vi "test Diff Configuration (Add Remove Ports and Acyclic Frame).vi"(8 "error in":errorcluster, 11 "TestCase in":refnum<class "Refresh.lvclass">) -> (0 "error out":errorcluster, 3 "TestCase out":refnum<class "Refresh.lvclass">)   [LabVIEW 2020, in "Refresh.lvclass"]
uses:
  Refresh.lvclass
  <vilib>/addons/_JKI Toolkits/VI Tester/TestCase.llb/TestCase.lvclass
  System Explorer/Implementation/System Explorer/Refresh/Refresh.lvlib
  Shared/Parameter Definition.ctl
  Shared/Address.ctl
  Shared/Terminal Endpoint.ctl
  Shared/Message Type.ctl
  Shared/Message Definition.ctl
  Shared/1553 Channel.ctl
  System Explorer/Implementation/System Explorer/Refresh/Symbols.ctl
  System Explorer/Implementation/System Explorer/Refresh/Change Type.ctl
  System Explorer/Implementation/System Explorer/Refresh/MCL Row.ctl
  C:/Program Files (x86)/National Instruments/LabVIEW 2020/vi.lib/addons/_JKI Toolkits/VI Tester/TestCase.llb/TestCase.lvclass
panel:
  out "Multicolumn Listbox":i32(listbox)=-1
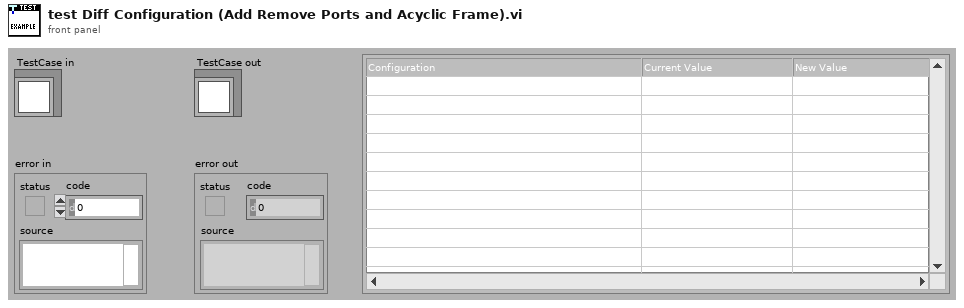
[diagram p1: front panel]
types:
  T1 = typedef "1553 Channel.ctl" = cluster{"HW channel":u16, "bus controller":cluster{"simulated?":bool, "name":string}, "terminal addresses":T2[], "terminal names":string[], "acyclic frame names":string[], "messages":T3[]}
  T2 = typedef "Address.ctl" = u16
  T3 = typedef "Message Definition.ctl" = cluster{"name":string, "message type":T4, "endpoint Tx":T5, "endpoint Rx":T5, "create timestamp channel":bool, "mode code":u16, "number of words":u16, "parameters":cluster{"name":string, "default value":dbl, "unit":string, "parameter definition":T6}[]}
  T4 = typedef "Message Type.ctl" = string
  T5 = typedef "Terminal Endpoint.ctl" = cluster{"terminal address":T2, "subaddress":T2}
  T6 = typedef "Parameter Definition.ctl" = cluster{"start index":i32, "size (bits)":i32, "encoding":enum16{"BNR", "BCD", "Discrete"}, "signed":bool, "multiplier":dbl, "offset":dbl}
  T7 = typedef "Ballard MIL-STD-1553 System Explorer.lvlib/Implementation.lvlib/Refresh.lvlib/MCL Row.ctl" = cluster{"change type":T8, "item symbol":T9, "item names":string[]}
  T8 = typedef "Ballard MIL-STD-1553 System Explorer.lvlib/Implementation.lvlib/Refresh.lvlib/Change Type.ctl" = enum16{"No change", "Modify", "Add", "Remove"}
  T9 = typedef "Ballard MIL-STD-1553 System Explorer.lvlib/Implementation.lvlib/Refresh.lvlib/Symbols.ctl" = enum16{"Blank", "MIL-STD-1553", "Port", "Remote Terminal", "Subaddress", "Bus Controller", "Acyclic Frame", "Mode Code", "Message", "Parameter", "Item"}
  T10 = typedef "imagedata.ctl" = cluster{"image type":i32, "image depth":i32, "image":u8[], "mask":u8[], "colors":u32[], "Rectangle":cluster{"left":i16, "top":i16, "right":i16, "bottom":i16}}
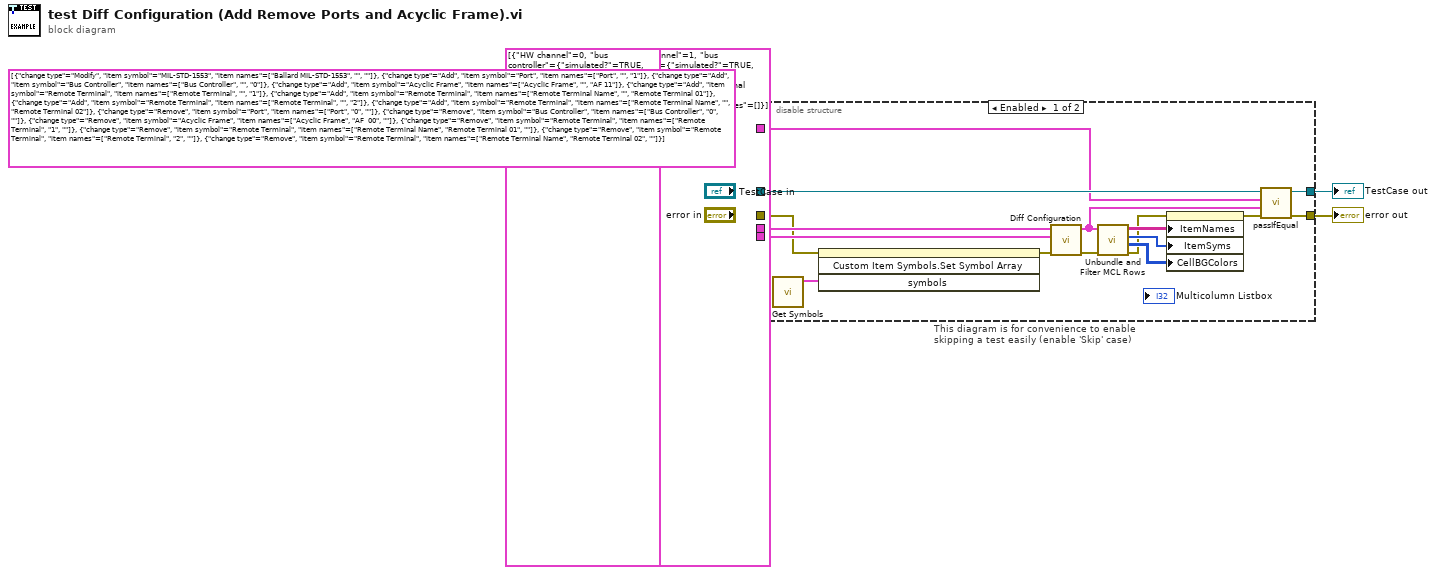
[diagram p0: block diagram]
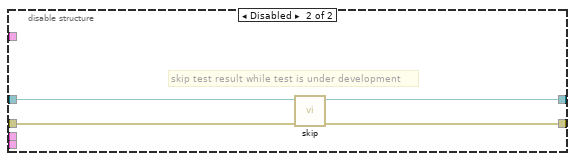
[diagram p2: hidden frame]
diagram:
  n1 = disable-structure "This diagram is for convenience to enable skipping a test easily (enable 'Skip' case)" shown="Enabled" {
    disable-tunnel: "TestCase in" -> [w23 w27]
    disable-tunnel: [w22 w25] -> w4
    disable-tunnel: [w8 w26] -> w6
    disable-tunnel: "error in" -> [w14 w24]
    disable-tunnel: T1[] [{"HW channel"=0, "bus controller"={"simulated?"=TRUE, "name"=""}, "terminal addresses"=[0, 1, 2], "terminal names"=[], "acyclic frame names"=["AF  00"], "messages"=[]}] -> [w21 _]
    disable-tunnel: T1[] [{"HW channel"=1, "bus controller"={"simulated?"=TRUE, "name"=""}, "terminal addresses"=[0, 1, 2], "terminal names"=[], "acyclic frame names"=["AF 11"], "messages"=[]}] -> [w20 _]
    disable-tunnel: T7[] [{"change type"=enum."Modify", "item symbol"=enum."MIL-STD-1553", "item names"=["Ballard MIL-STD-1553", "", ""]}, {"change type"=enum."Add", "item symbol"=enum."Port", "item names"=["Port", "", "1"]}, {"change type"=enum."Add", "item symbol"=enum."Bus Controller", "item names"=["Bus Controller", "", "0"]}, {"change type"=enum."Add", "item symbol"=enum."Acyclic Frame", "item names"=["Acyclic Frame", "", "AF 11"]}, {"change type"=enum."Add", "item symbol"=enum."Remote Terminal", "item names"=["Remote Terminal", "", "1"]}, {"change type"=enum."Add", "item symbol"=enum."Remote Terminal", "item names"=["Remote Terminal Name", "", "Remote Terminal 01"]}, {"change type"=enum."Add", "item symbol"=enum."Remote Terminal", "item names"=["Remote Terminal", "", "2"]}, {"change type"=enum."Add", "item symbol"=enum."Remote Terminal", "item names"=["Remote Terminal Name", "", "Remote Terminal 02"]}, {"change type"=enum."Remove", "item symbol"=enum."Port", "item names"=["Port", "0", ""]}, {"change type"=enum."Remove", "item symbol"=enum."Bus Controller", "item names"=["Bus Controller", "0", ""]}, {"change type"=enum."Remove", "item symbol"=enum."Acyclic Frame", "item names"=["Acyclic Frame", "AF  00", ""]}, {"change type"=enum."Remove", "item symbol"=enum."Remote Terminal", "item names"=["Remote Terminal", "1", ""]}, {"change type"=enum."Remove", "item symbol"=enum."Remote Terminal", "item names"=["Remote Terminal Name", "Remote Terminal 01", ""]}, {"change type"=enum."Remove", "item symbol"=enum."Remote Terminal", "item names"=["Remote Terminal", "2", ""]}, {"change type"=enum."Remove", "item symbol"=enum."Remote Terminal", "item names"=["Remote Terminal Name", "Remote Terminal 02", ""]}] ("configuration diff") -> [w11 _]
    frame Enabled {
      n2 = call "Get Symbols.vi"() -> ("MIL-STD-1553 symbols"=w15:T10[])  [unwired: 11 in]
      n3 = invoke on="Multicolumn Listbox" class="MCListbox (strict)" method="Custom Item Symbols.Set Symbol Array"(error in=w14, "symbols"=w15) -> (error out=w13:errorcluster)  [unwired: 2 in, 3 out]
      n4 = call "Diff Configuration.vi"("error in"=w13, "configuration new"=w20, "configuration old"=w21) -> ("error out"=w10:errorcluster, "configuration diff"=w12:T7[])  [unwired: 7 in]
      n5 = call "Unbundle and Filter MCL Rows.vi"("error in"=w10, "refresh items"=w12) -> ("error out"=w16:errorcluster, "background colors"=w19:u32[][], "item symbols"=w18:T9[], "item names"=w17:string[][])  [unwired: 6 in]
      n6 = property on="Multicolumn Listbox" class="MCListbox (strict)"(error in=w16, "ItemNames"=w17, "ItemSyms"=w18, "CellBGColors"=w19) -> (error out=w9:errorcluster)  [unwired: 1 in, 1 out]
      n7 = call-dynamic "passIfEqual.vi"("error in (no error)"=w9, "y"=w12, "x"=w11, "TestCase in"=w23) -> ("error out"=w8:errorcluster, "TestCase out"=w22:refnum<class "Refresh.lvclass">)  [unwired: 6 in]
    }
    frame Disabled {
      # "skip test result while test is under development"
      n8 = call <vilib>:"skip.vi"("error in (no error)"=w24, "TestCase in"=w27) -> ("error out"=w26:errorcluster, "TestCase out"=w25:refnum<class "Refresh.lvclass">)  [unwired: 8 in]
    }
  }
  "error out" <- w6
  "TestCase out" <- w4
